vi "includePhysicalChannelsIntoData.vi"(8 "error in (no error)":errorcluster, 10 "Data":T1={"Timestamps ms"=[0.0, 0.005, 0.009, 0.012], "DataPerChannel"=[]} {"Timestamps ms" format="%.3f"}, 11 "DIO64Output in":refnum<class "DIO64Output.lvclass">) -> (0 "error out":errorcluster, 2 "Data out":T1, 3 "DIO64Output out":refnum<class "DIO64Output.lvclass">)   [LabVIEW 2011, in "Hardware.lvlib" / "Channels.lvlib" / "DIO64Output.lvclass"]
uses:
  DIO64Output.lvclass
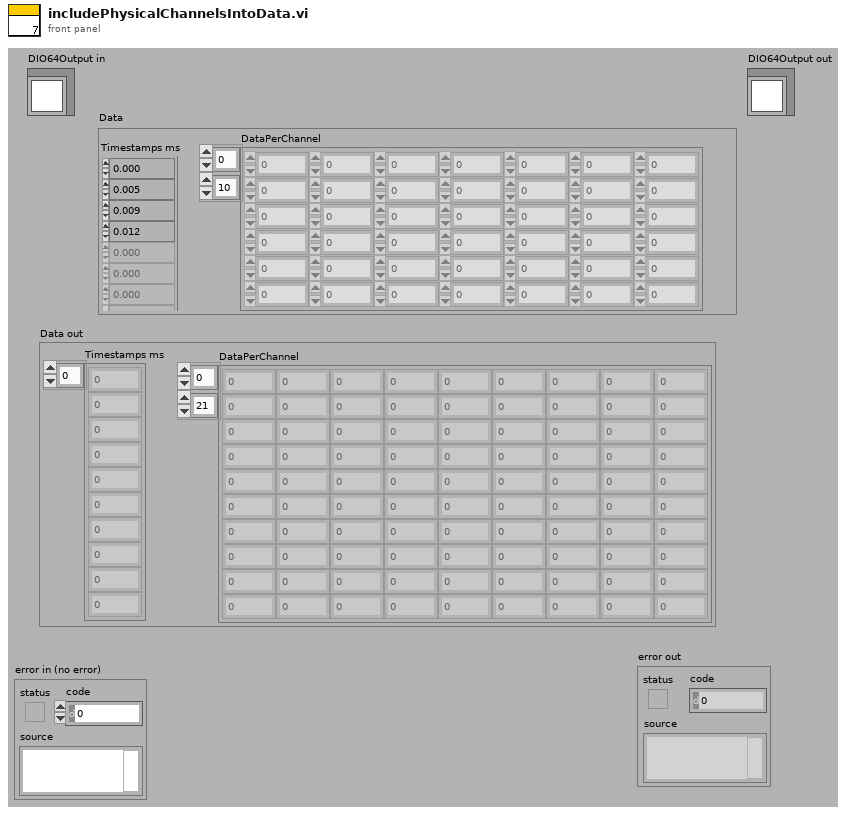
[diagram p1: front panel]
types:
  T1 = cluster{"Timestamps ms":dbl[], "DataPerChannel":dbl[][]}
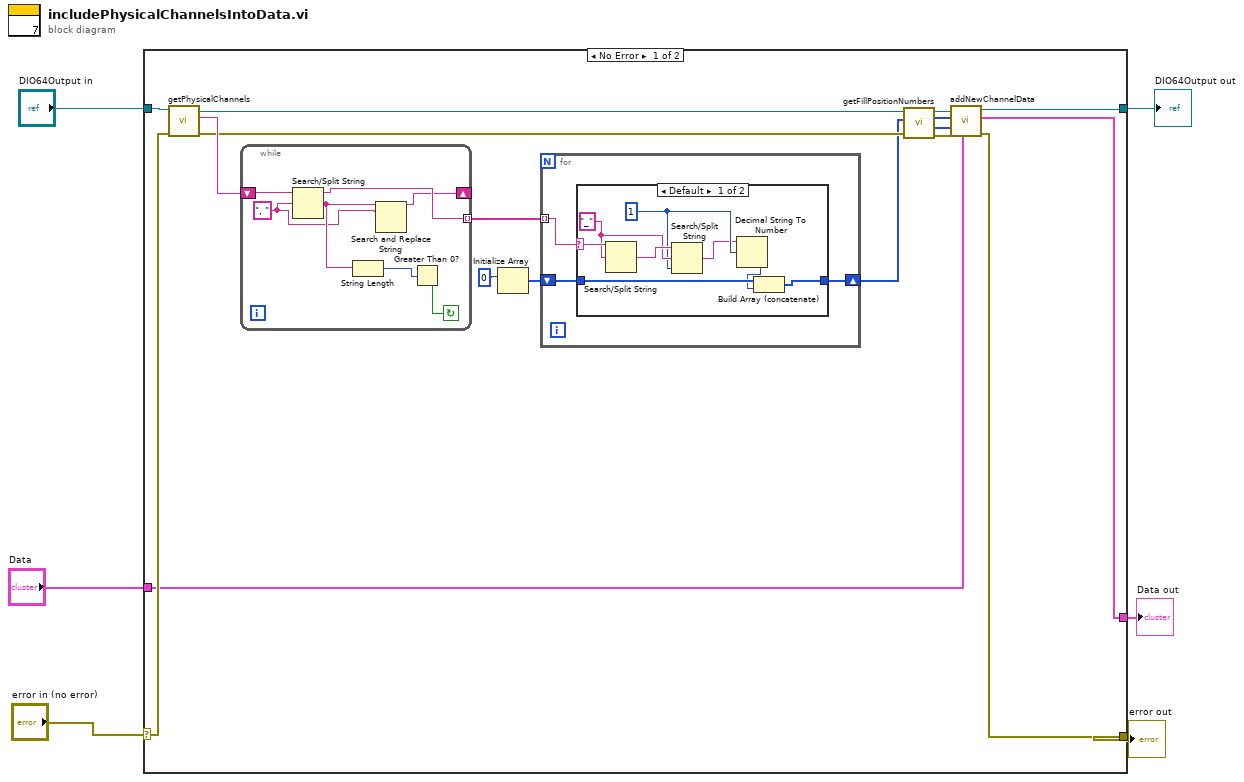
[diagram p0: block diagram]
diagram:
  n1 = case shown="No Error" "error in (no error)" {
    selector: "error in (no error)" -> [w22 w44]
    tunnel: [w8 w44] -> w5
    tunnel: [w9 w43] -> w3
    tunnel: "DIO64Output in" -> [w23 w43]
    tunnel: "Data" -> [w10 _]
    tunnel: [w7 _] -> w1
    frame No Error {
      n2 = call-dynamic "getPhysicalChannels.vi"("error in (no error)"=w22, "DigitalOutput.lvclass in"=w23) -> ("error out"=w12:errorcluster, "Physical Channels"=w21:string, "DigitalOutput.lvclass out"=w13:refnum<class "DIO64Output.lvclass">)  [unwired: 7 in]
      n3 = while {
        shift-right: [w38] -> _
        shift-left: w21 -> [w42]
        tunnel: [w41] -> w20 mode=indexing
        stop <- w36 continue-if-true
        w39 = ", "
        n4 = Search/Split String(string=w42, search string/char (-)=w39) -> (substring before match=w41:string, match + rest of string=w40:string)  [unwired: 1 in, 1 out]
        n5 = String Length(string=w40) -> (length=w37:i32)
        n6 = Search and Replace String(input string=w40, search string=w39) -> (result string=w38:string)  [unwired: 6 in, 3 out]
        n7 = Greater Than 0?(x=w37) -> (x > 0?=w36:bool)
      }
      n8 = Initialize Array(0) -> (w19:i32[])  [unwired: 1 in]
      n9 = for {
        tunnel: w20 -> [w26] mode=indexing
        shift-right: [w24] -> w11
        shift-left: w19 -> [w25]
        n10 = case shown="Default" w26 {
          selector: w26 -> [w31 _]
          tunnel: w25 -> [w34 w35]
          tunnel: [w32 w35] -> w24
          frame Default {
            w28 = 1
            w29 = "_"
            n11 = Search/Split String(string=w31, search string/char (-)=w29) -> (match + rest of string=w30:string)  [unwired: 1 in, 2 out]
            n12 = Search/Split String(string=w30, search string/char (-)=w29, offset (0)=w28) -> (match + rest of string=w27:string)  [unwired: 2 out]
            n13 = Decimal String To Number(string=w27, offset=w28) -> (number=w33:i32)  [unwired: 1 in, 1 out]
            n14 = Build Array (concatenate)(w34, w33) -> (w32:i32[])
          }
          frame "" {
          }
        }
      }
      n15 = call "getFillPositionNumbers.vi"("error in (no error)"=w12, "Array"=w11, "DIO64Output in"=w13) -> ("error out"=w14:errorcluster, "fill number"=w15:i32[], "position"=w16:i32[], "DIO64Output out"=w17:refnum<class "DIO64Output.lvclass">)  [unwired: 5 in]
      n16 = call "addNewChannelData.vi"("Data In"=w10, "error in (no error)"=w14, "fill number"=w15, "position"=w16, "DIO64Output in"=w17) -> ("error out"=w8:errorcluster, "Dataout"=w7:T1, "DIO64Output out"=w9:refnum<class "DIO64Output.lvclass">)  [unwired: 4 in]
    }
    frame Error {
    }
  }
  "error out" <- w5
  "DIO64Output out" <- w3
  "Data out" <- w1
